vi "Add.vi"(10 "B":dbl, 11 "A":dbl) -> (3 "Result":dbl(knob) scale=0.0..10.0)   [LabVIEW 2024]
doc: "Adds two numbers together and returns the result."
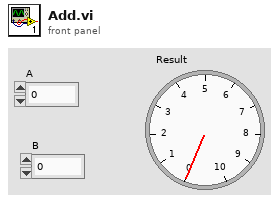
[diagram p1: front panel]
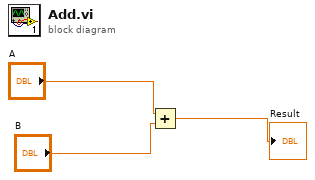
[diagram p0: block diagram]
diagram:
  n1 = Add(x="A", y="B") -> (x+y=→"Result":dbl)
